vi "Stop Core.vi"(10 "final error code":i32, 11 "Transfer Line in":refnum<class "Transfer Line.lvclass">) -> (3 "Transfer Line out":refnum<class "Transfer Line.lvclass">)   [LabVIEW 2015, in "cRIO-Carbondioxide.lvlib" / "CO2-Actor.lvlib" / "Transfer Line.lvclass"]
doc: "(<B>Filename</B>: Actor Framework.lvlib:Actor.lvclass:Stop Core.vi)\n\nDefines what the actor does before it stops. Use the <B>final error code</B> input to determine whether the actor shut down in response to an error.\n\nBy default, this method does nothing. A descendant class may override it to define behavior, such as shutting down any processes the actor initiated in its override of the Actor Core method."
uses:
  Transfer Line.lvclass
  Transfer Line.lvclass/Transfer Line.ctl
  CO2 Actor/CO2 Actor.lvclass
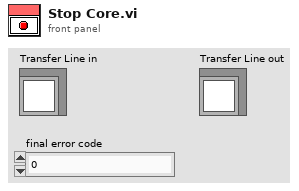
[diagram p1: front panel]
types:
  T1 = typedef "Sample Container.ctl" = cluster{"Sample In":refnum<k21>, "Sample Name":refnum<k21>, "Ti Cathode":refnum<k21>, "SampleQ":refnum<queue>}
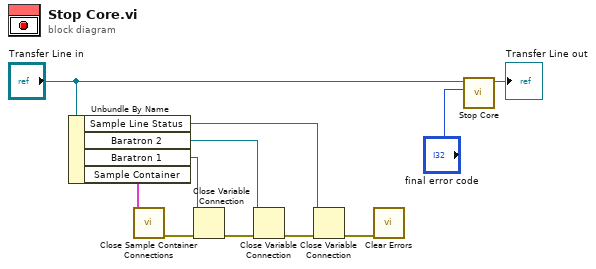
[diagram p0: block diagram]
diagram:
  n1 = Unbundle By Name("Transfer Line in") -> ("Sample Line Status"=w5:refnum<k21>, "Baratron 2"=w6:refnum<k21>, "Baratron 1"=w7:refnum<k21>, "Sample Container"=w8:T1)
  n2 = call "Close Sample Container Connections.vi"("Container in"=w8) -> ("error out"=w4:errorcluster)  [unwired: 9 in, 1 out]
  n3 = Close Variable Connection(8:w4, 11:w7) -> (0:w3:errorcluster)
  n4 = Close Variable Connection(8:w3, 11:w6) -> (0:w2:errorcluster)
  n5 = Close Variable Connection(8:w2, 11:w5) -> (0:w1:errorcluster)
  n6 = call <vilib>:"Clear Errors.vi"("error in (no error)"=w1) -> ()  [unwired: 5 in, 2 out]
  n7 = call-parent "Stop Core.vi"("final error code"="final error code", "CO2 Actor in"="Transfer Line in") -> ("CO2 Actor out"=→"Transfer Line out":refnum<class "Transfer Line.lvclass">)  [unwired: 9 in]
